vi "SetArmState.vi"(8 "error in":errorcluster, 11 "ArmState":enum16{"Up", "Down"}(ring)) -> (0 "error out":errorcluster)   [LabVIEW 2016]
doc: "Sets arm state global variable"
uses:
  Robot Global Data.vi
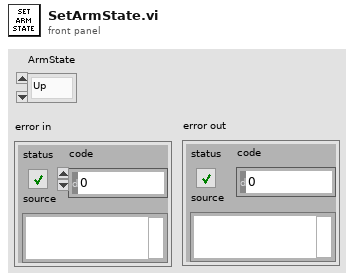
[diagram p1: front panel]
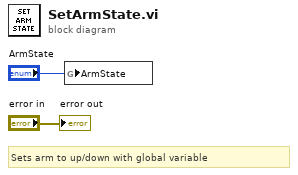
[diagram p0: block diagram]
diagram:
  # "Sets arm to up/down with global variable"
  n1 = global write "Robot Global Data.vi" "ArmState"("ArmState") -> ()
  "error out" <- "error in"
